vi "Launcher.vi"() -> ()   [LabVIEW 2024]
uses:
  <vilib>/Utility/miscctls.llb/LVRectTypeDef.ctl
  <vilib>/numeric/sub_Random U32.vi
  Logger/Logger.lvclass
  C:/Users/burakkorkmaz/Desktop/Leveling/labview-design-patterns/Observer Pattern/IObserver/IObserver.lvclass
  Controller/Controller.lvclass
  CommunicationModule/CommunicationModule.lvclass
  <vilib>/numeric/Random Number (Range) U64.vi
  C:/Users/burakkorkmaz/Desktop/Leveling/labview-design-patterns/Observer Pattern/Controller/Controller.lvclass
  C:/Users/burakkorkmaz/Desktop/Leveling/labview-design-patterns/Observer Pattern/Logger/Logger.lvclass
panel:
  out "error out":errorcluster
  out "Random Number":string
  in  "Stop":bool
  out "CONTROLLER":string
  out "LOGGER":string
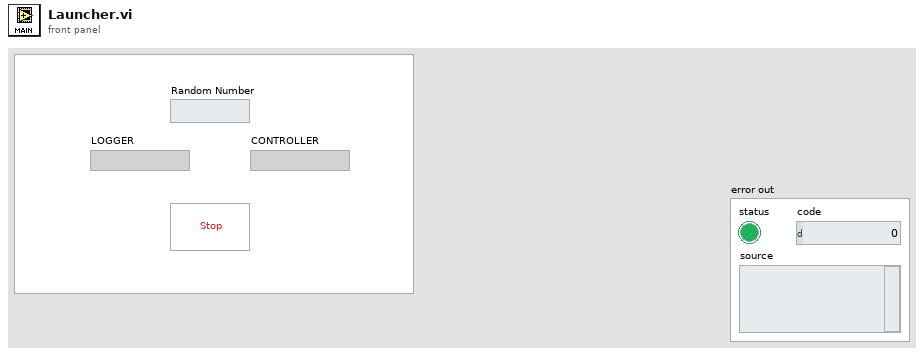
[diagram p1: front panel]
types:
  T1 = typedef "LVRectTypeDef.ctl" = cluster{"Left":i16, "Top":i16, "Right":i16, "Bottom":i16}
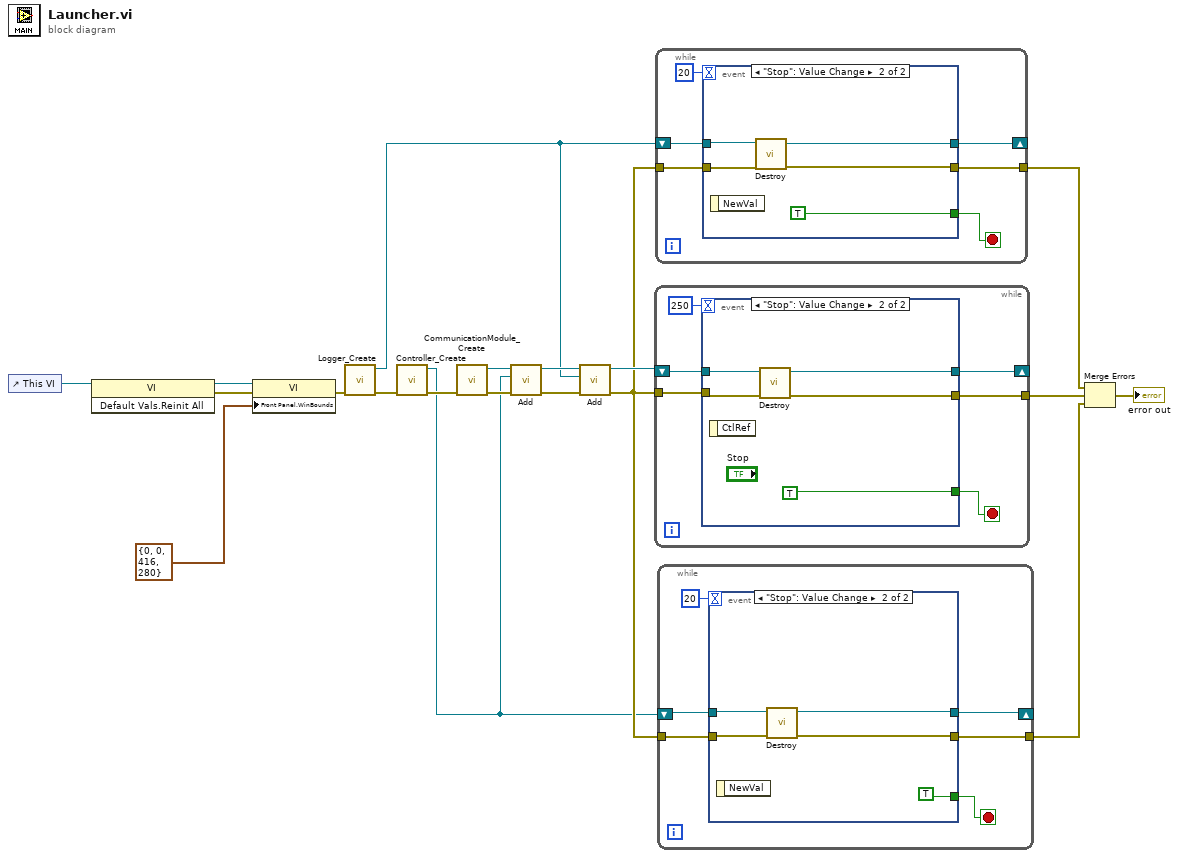
[diagram p0: block diagram]
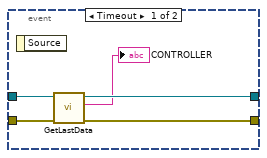
[diagram p2: hidden frame]
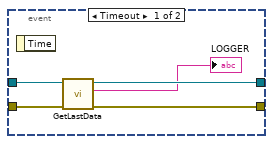
[diagram p3: hidden frame]
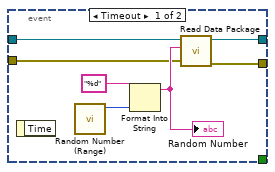
[diagram p4: hidden frame]
diagram:
  n1 = control-ref of="This VI"() -> (w14:refnum<vi>)
  n2 = invoke class="VI" method="Default Vals.Reinit All"(reference=w14) -> (reference out=w2:refnum<vi>, error out=w13:errorcluster)  [unwired: 2 in, 1 out]
  n3 = property class="VI"(reference=w2, error in=w13, "Front Panel.WinBounds"=T1 {"Left"=0, "Top"=0, "Right"=416, "Bottom"=280} ("Front Panel Window:Window Bounds")) -> (error out=w3:errorcluster)  [unwired: 1 out]
  n4 = call "Logger_Create.vi"("Error In"=w3) -> ("Error Out"=w11:errorcluster, "reference out"=w8:refnum<class "Logger.lvclass">)  [unwired: 9 in]
  n5 = call "Controller_Create.vi"("Error In"=w11) -> ("Error Out"=w10:errorcluster, "reference out"=w9:refnum<class "Controller.lvclass">)  [unwired: 9 in]
  n6 = call "CommunicationModule_Create.vi"("Error In"=w10) -> ("Error Out"=w12:errorcluster, "reference out"=w19:refnum<class "CommunicationModule.lvclass">)  [unwired: 9 in]
  n7 = call-dynamic "Add.vi"("Error In"=w12, "IObserver"=w9, "reference in"=w19) -> ("Error Out"=w16:errorcluster, "reference out"=w18:refnum<class "CommunicationModule.lvclass">)  [unwired: 7 in]
  n8 = call-dynamic "Add.vi"("Error In"=w16, "IObserver"=w8, "reference in"=w18) -> ("Error Out"=w15:errorcluster, "reference out"=w17:refnum<class "CommunicationModule.lvclass">)  [unwired: 7 in]
  n9 = while {
    tunnel: w15 -> [w23]
    tunnel: [w22] -> w6
    shift-right: [w24] -> _
    shift-left: w17 -> [w25]
    stop <- w21 stop-if-true
    n10 = event shown="[1] \"Stop\": Value Change" {
      selector: _ -> [_ _]
      dyn-events: _ -> [_ _]
      timeout: 250 -> [_ _]
      tunnel: w25 -> [w32 w33]
      tunnel: [w28 w35] -> w24
      tunnel: w23 -> [w27 w34]
      tunnel: [w26 w36] -> w22
      tunnel: [_ TRUE] -> w21
      event Timeout {
        n11 = event-data() -> ()  [unwired: 1 in, 1 out]
        n12 = call-poly <vilib>:"Random Number (Range).vi"() -> ("number"=w31:u64)  [unwired: 11 in]
        n13 = Format Into String(format string="%d", w31) -> (resulting string=w29:string)  [unwired: 2 in, 1 out]
        "Random Number" <- w29
        n14 = call "Read Data Package.vi"("Error In"=w27, "Data"=w29, "reference in"=w32) -> ("Error Out"=w26:errorcluster, "reference out"=w28:refnum<class "CommunicationModule.lvclass">)  [unwired: 7 in]
      }
      event "Stop": Value Change {
        n15 = event-data() -> ()  [unwired: 1 in, 1 out]
        n16 = call-dynamic "Destroy.vi"("Error In"=w34, "reference in"=w33) -> ("Error Out"=w36:errorcluster, "reference out"=w35:refnum<class "CommunicationModule.lvclass">)  [unwired: 8 in]
      }
    }
  }
  n17 = while {
    tunnel: w15 -> [w42]
    tunnel: [w41] -> w7
    shift-right: [w40] -> _
    shift-left: w8 -> [w43]
    stop <- w38 stop-if-true
    n18 = event shown="[1] \"Stop\": Value Change" {
      selector: _ -> [_ _]
      dyn-events: _ -> [_ _]
      timeout: 20 -> [_ _]
      tunnel: w43 -> [w48 w50]
      tunnel: w42 -> [w47 w49]
      tunnel: [w46 w52] -> w41
      tunnel: [w45 w51] -> w40
      tunnel: [_ TRUE] -> w38
      event Timeout {
        n19 = event-data() -> ()  [unwired: 1 in, 1 out]
        n20 = call-dynamic "GetLastData.vi"("Error In"=w47, "reference in"=w48) -> ("Error Out"=w46:errorcluster, "LastData"=→"LOGGER":string, "reference out"=w45:refnum<class "Logger.lvclass">)  [unwired: 7 in]
      }
      event "Stop": Value Change {
        n21 = event-data() -> ()  [unwired: 1 in, 1 out]
        n22 = call-dynamic "Destroy.vi"("Error In"=w49, "reference in"=w50) -> ("Error Out"=w52:errorcluster, "reference out"=w51:refnum<class "Logger.lvclass">)  [unwired: 8 in]
      }
    }
  }
  n23 = while {
    tunnel: w15 -> [w58]
    tunnel: [w56] -> w5
    shift-right: [w57] -> _
    shift-left: w9 -> [w59]
    stop <- w54 stop-if-true
    n24 = event shown="[1] \"Stop\": Value Change" {
      selector: _ -> [_ _]
      dyn-events: _ -> [_ _]
      timeout: 20 -> [_ _]
      tunnel: w59 -> [w64 w66]
      tunnel: w58 -> [w63 w65]
      tunnel: [w62 w67] -> w57
      tunnel: [w61 w68] -> w56
      tunnel: [_ TRUE] -> w54
      event Timeout {
        n25 = event-data() -> ()  [unwired: 1 in, 1 out]
        n26 = call-dynamic "GetLastData.vi"("Error In"=w63, "reference in"=w64) -> ("Error Out"=w61:errorcluster, "LastData"=→"CONTROLLER":string, "reference out"=w62:refnum<class "Controller.lvclass">)  [unwired: 7 in]
      }
      event "Stop": Value Change {
        n27 = event-data() -> ()  [unwired: 1 in, 1 out]
        n28 = call-dynamic "Destroy.vi"("Error In"=w65, "reference in"=w66) -> ("Error Out"=w68:errorcluster, "reference out"=w67:refnum<class "Controller.lvclass">)  [unwired: 8 in]
      }
    }
  }
  n29 = Merge Errors(w7, w6, w5) -> (→"error out":errorcluster)
